vi "initialize action with configuration.vi"(8 "error in (no error)":errorcluster, 9 "action configuration":refnum<class "action configuration.lvclass">, 10 "sequencer data allocations":T1, 11 "Simple Sequencer TBM configuration in":refnum<class "Simple Sequencer TBM configuration.lvclass">) -> (0 "error out":errorcluster, 1 "actions with configuration out":T4, 2 "sequencer data allocations out":T1, 3 "Simple Sequencer TBM configuration out":refnum<class "Simple Sequencer TBM configuration.lvclass">)   [LabVIEW 2014, in "Simple Sequencer TBM runtime.lvclass"]
doc: "Initializes an action and the data space (parameters and results) for data exchanged with that action."
uses:
  Simple Sequencer TBM runtime.lvclass
  configuration/Simple Sequencer TBM configuration.lvclass
  sequencer parent classes/action configuration parent/action configuration.lvclass
  actions with configuration.ctl
  sequencer parent classes/action parent/action.lvclass
  <vilib>/NI/Tag Bus/table/data table.ctl
  <vilib>/NI/Tag Bus/table/transfer specification.ctl
  <vilib>/NI/Tag Bus/tag/Data Type.ctl
  <vilib>/NI/Tag Bus Module Framework/channel/data tables.ctl
  <vilib>/NI/Tag Bus/dictionary/data dictionary.lvclass
  <vilib>/NI/Tag Bus/dictionary table pair.ctl
  <vilib>/NI/Configuration Framework/serializable configuration/NISE_CEF_serializable configuration.lvclass/NISE_CEF_serializable configuration.ctl
  <vilib>/NI/Configuration Framework/serializable configuration/Read UID.vi
  <vilib>/Utility/LVClass/Get LV Class Name.vi
  <vilib>/NI/Configuration Framework/error generator/NISE_error generator.vi
  sequencer parent classes/sequencer config parent/base TBM sequencer configuration.lvclass
  <vilib>/NI/Tag Bus/tag/tag descriptor.lvclass
  <vilib>/NI/Tag Bus/table/data table.lvlib
  <vilib>/NI/Tag Bus/tag bus.lvlib
  <vilib>/NI/Tag Bus Module Framework/channel/TBM channel.lvclass
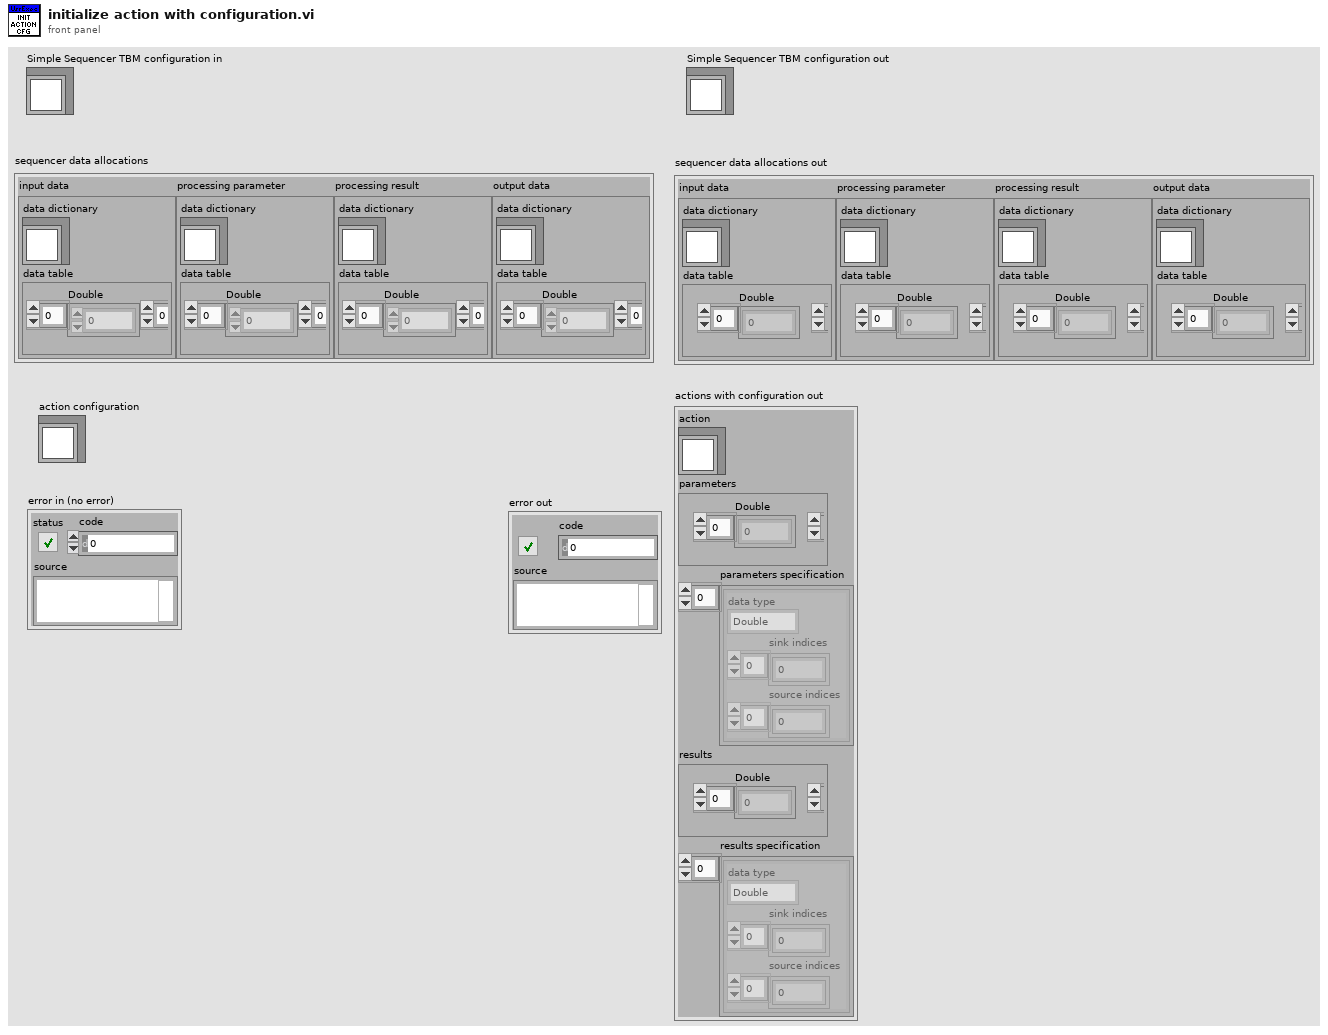
[diagram p1: front panel]
types:
  T1 = typedef "TBM channel.lvclass/data tables.ctl" = cluster{"input data":T2, "processing parameter":T2, "processing result":T2, "output data":T2}
  T2 = typedef "tag bus.lvlib/dictionary table pair.ctl" = cluster{"data dictionary":refnum<class "data dictionary.lvclass">, "data table":T3}
  T3 = typedef "tag bus.lvlib/data table.lvlib/data table.ctl" = cluster{"Double":dbl[], "Single":sgl[], "I64":i64[], "I32":i32[], "I16":i16[], "I8":i8[], "U64":u64[], "U32":u32[], "U16":u16[], "U8":u8[], "Boolean":bool[], "String":string[], "Array of Double":cluster{"DBL Array":dbl[]}[], "Array of Single":cluster{"SGL Array":sgl[]}[], "Array of I64":cluster{"I64 Array":i64[]}[], "Array of I32":cluster{"I32 Array":i32[]}[], "Array of I16":cluster{"I16 Array":i16[]}[], "Array of I8":cluster{"I8 Array":i8[]}[], "Array of U64":cluster{"U64 Array":u64[]}[], "Array of U32":cluster{"U32 Array":u32[]}[], "Array of U16":cluster{"U16 Array":u16[]}[], "Array of U8":cluster{"U8 Array":u8[]}[], "Array of Boolean":cluster{"Boolean Array":bool[]}[], "Array of String":cluster{"String Array":string[]}[]}
  T4 = typedef "Simple Sequencer TBM runtime.lvclass/actions with configuration.ctl" = cluster{"action":refnum<class "action.lvclass">, "parameters":T3, "parameters specification":T5[], "results":T3, "results specification":T5[]}
  T5 = typedef "tag bus.lvlib/data table.lvlib/transfer specification.ctl" = cluster{"data type":T6, "sink indices":i32[], "source indices":i32[]}
  T6 = typedef "tag bus.lvlib/tag descriptor.lvclass/Data Type.ctl" = enum16{"Double", "Single", "I64", "I32", "I16", "I8", "U64", "U32", "U16", "U8", "Boolean", "String", "Array of Double", "Array of Single", "Array of I64", "Array of I32", "Array of I16", "Array of I8", "Array of U64", "Array of U32", "Array of U16", "Array of U8", "Array of Boolean", "Array of String"}
  T7 = typedef "base TBM sequencer configuration.lvclass/Module Mappings.ctl" = cluster{"Owning ID":string, "Input Mappings":T8[], "Process Parameter Mappings":T8[], "Process Results Mappings":T8[], "Output Mappings":T8[]}
  T8 = typedef "tag bus.lvlib/data table.lvlib/mapping specification.ctl" = cluster{"data type":T6, "mappings":T9[]}
  T9 = typedef "tag bus.lvlib/data table.lvlib/mapping.ctl" = cluster{"sink name":string, "source name":string}
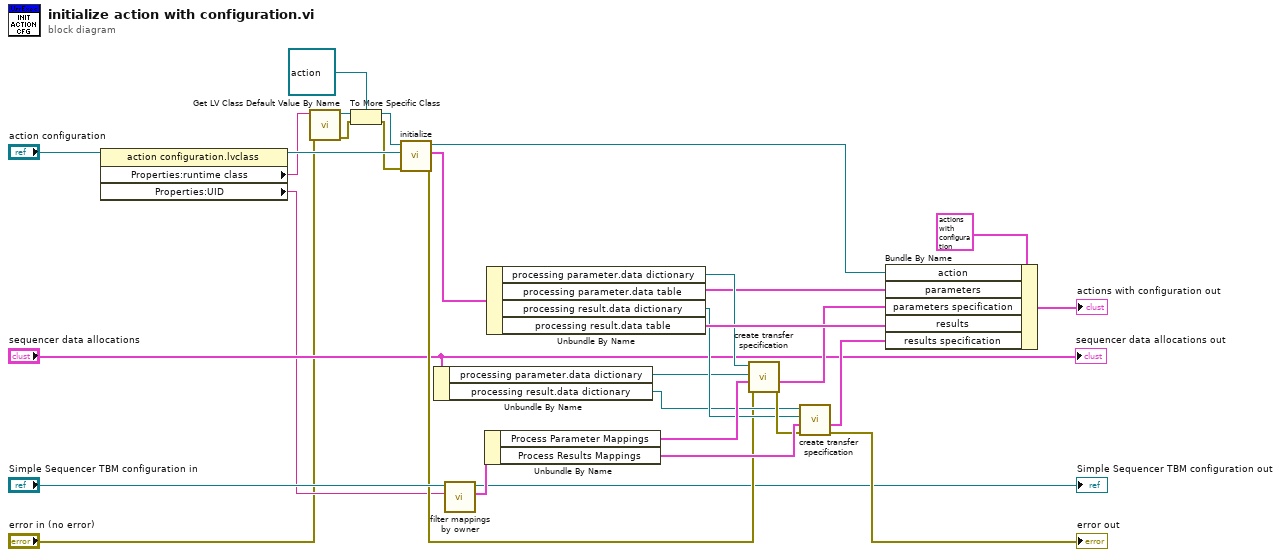
[diagram p0: block diagram]
diagram:
  n1 = property class="action configuration.lvclass"(reference="action configuration") -> (reference out=w14:refnum<class "action configuration.lvclass">, "Properties:runtime class"=w7:string, "Properties:UID"=w8:string)  [unwired: 1 in, 1 out]
  n2 = call <vilib>:"Get LV Class Default Value By Name.vi"("error in (no error)"="error in (no error)", "class name"=w7) -> ("error out"=w3:errorcluster, "object"=w4:refnum<class>)  [unwired: 8 in]
  n3 = To More Specific Class(target class=refnum<class "action.lvclass"> refnum ("Action in"), reference=w4, error in=w3) -> (specific class reference=w1:refnum<class "action.lvclass">, error out=w2:errorcluster)
  n4 = call-dynamic "initialize.vi"("error in (no error)"=w2, "action configuration"=w14, "Action in"=w1) -> ("error out"=w11:errorcluster, "data allocations"=w13:T1, "Action out"=w12:refnum<class "action.lvclass">)  [unwired: 6 in]
  n5 = Unbundle By Name("sequencer data allocations") -> ("processing parameter.data dictionary"=w18:refnum<class "data dictionary.lvclass">, "processing result.data dictionary"=w17:refnum<class "data dictionary.lvclass">)
  n6 = call "filter mappings by owner.vi"("owner"=w8, "engine configuration in"="Simple Sequencer TBM configuration in") -> ("module mapping"=w29:T7, "engine configuration out"=→"Simple Sequencer TBM configuration out":refnum<class "Simple Sequencer TBM configuration.lvclass">)  [unwired: 8 in]
  n7 = Unbundle By Name(w29) -> ("Process Parameter Mappings"=w30:T8[], "Process Results Mappings"=w31:T8[])
  n8 = Unbundle By Name(w13) -> ("processing parameter.data dictionary"=w21:refnum<class "data dictionary.lvclass">, "processing parameter.data table"=w20:T3, "processing result.data dictionary"=w23:refnum<class "data dictionary.lvclass">, "processing result.data table"=w26:T3)
  n9 = call <vilib>:"create transfer specification.vi"("error in"=w11, "mapping specification"=w30, "data dictionary source in"=w18, "data dictionary sink in"=w21) -> ("error out"=w24:errorcluster, "transfer specification"=w22:T5[])  [unwired: 4 in, 2 out]
  n10 = call <vilib>:"create transfer specification.vi"("error in"=w24, "mapping specification"=w31, "data dictionary source in"=w23, "data dictionary sink in"=w17) -> ("error out"=→"error out":errorcluster, "transfer specification"=w27:T5[])  [unwired: 4 in, 2 out]
  n11 = Bundle By Name(cluster=T4 {"action"=refnum, "parameters"={"Double"=[], "Single"=[], "I64"=[], "I32"=[], "I16"=[], "I8"=[], "U64"=[], "U32"=[], "U16"=[], "U8"=[], "Boolean"=[], "String"=[], "Array of Double"=[], "Array of Single"=[], "Array of I64"=[], "Array of I32"=[], "Array of I16"=[], "Array of I8"=[], "Array of U64"=[], "Array of U32"=[], "Array of U16"=[], "Array of U8"=[], "Array of Boolean"=[], "Array of String"=[]}, "parameters specification"=[], "results"={"Double"=[], "Single"=[], "I64"=[], "I32"=[], "I16"=[], "I8"=[], "U64"=[], "U32"=[], "U16"=[], "U8"=[], "Boolean"=[], "String"=[], "Array of Double"=[], "Array of Single"=[], "Array of I64"=[], "Array of I32"=[], "Array of I16"=[], "Array of I8"=[], "Array of U64"=[], "Array of U32"=[], "Array of U16"=[], "Array of U8"=[], "Array of Boolean"=[], "Array of String"=[]}, "results specification"=[]} ("actions with configuration"), "action"=w12, "parameters"=w20, "parameters specification"=w22, "results"=w26, "results specification"=w27) -> (→"actions with configuration out":T4)
  "sequencer data allocations out" <- "sequencer data allocations"
